vi "Write Message.vi"(7 "Message Type":T1, 8 "timeout ms (5000)":i32=5000, 9 "String":string, 10 "error in (no error)":errorcluster, 11 "RawSocket Handler in":refnum<class "RawSocket Handler.lvclass">) -> (2 "error out":errorcluster, 3 "RawSocket Handler out":refnum<class "RawSocket Handler.lvclass">)   [LabVIEW 2020, in "wamplv.lvlib" / "RawSocket Handler.lvclass"]
uses:
  RawSocket Handler.lvclass
  Message Type.ctl
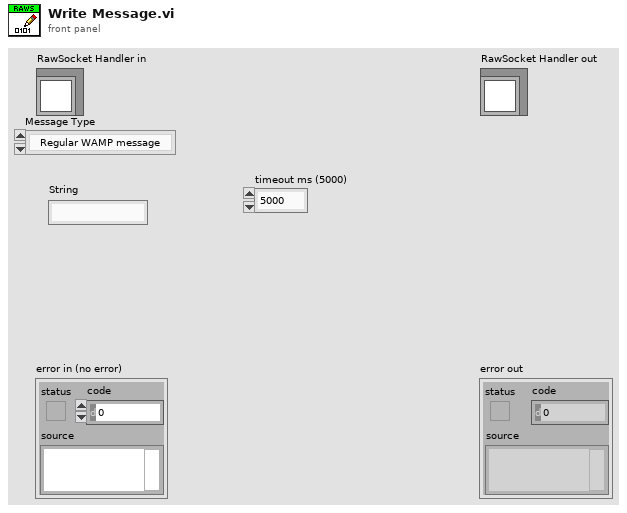
[diagram p1: front panel]
types:
  T1 = typedef "wamplv.lvlib/RawSocket Handler.lvclass/Message Type.ctl" = enum8{"Regular WAMP message", "PING", "PONG"}
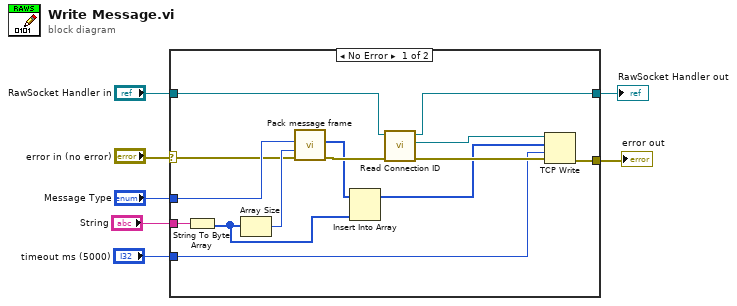
[diagram p0: block diagram]
diagram:
  n1 = case shown="No Error" "error in (no error)" {
    selector: "error in (no error)" -> [w16 w22]
    tunnel: "Message Type" -> [w21 _]
    tunnel: "String" -> [w20 _]
    tunnel: "RawSocket Handler in" -> [w15 w23]
    tunnel: [w14 w23] -> w3
    tunnel: "timeout ms (5000)" -> [w12 _]
    tunnel: [w11 w22] -> w1
    frame No Error {
      n2 = String To Byte Array(string=w20) -> (unsigned byte array=w9:u8[])
      n3 = Array Size(array=w9) -> (size(s)=w19:i32)
      n4 = call "Pack message frame.vi"("error in"=w16, "Size (bytes)"=w19, "Message Type"=w21) -> ("error out"=w18:errorcluster, "Message frame"=w10:u8[])  [unwired: 7 in]
      n5 = Insert Into Array(array=w10, new element=w9) -> (w8:u8[])  [unwired: 1 in]
      n6 = call-dynamic "Read Connection ID.vi"("error in (no error)"=w18, "RawSocket Handler in"=w15) -> ("error out"=w17:errorcluster, "Connection ID"=w13:refnum<k5>, "RawSocket Handler out"=w14:refnum<class "RawSocket Handler.lvclass">)  [unwired: 7 in]
      n7 = TCP Write(connection ID=w13, data in=w8, error in (no error)=w17, 9:w12) -> (error out=w11:errorcluster)  [unwired: 2 out]
    }
    frame Error {
    }
  }
  "error out" <- w1
  "RawSocket Handler out" <- w3
